vi "HART_init_address_and_MODBUS_register.vi"() -> ()   [LabVIEW 2016]
panel:
  out "Array":u16[](array[numeric])
  out "Floating pt.":sgl[](array[numeric])=[496.45227, -0.008102778, 0.0, 0.0, 0.0, 0.0, 0.0, 0.0]
  in  "Array of registers to read":T1(array[cluster])=[{"MODBUS Reg."=285, "data type"=enum."Float", "Desc."="Tube frequency"}, {"MODBUS Reg."=247, "data type"=enum."Float", "Desc."="Mass Flow"}, {"MODBUS Reg."=419, "data type"=enum."Uint16", "Desc."="Status word 1"}, {"MODBUS Reg."=420, "data type"=enum."Uint16", "Desc."="Status word 2"}, {"MODBUS Reg."=421, "data type"=enum."Uint16", "Desc."="Status word 3"}, {"MODBUS Reg."=422, "data type"=enum."Uint16", "Desc."="Status word 4"}, {"MODBUS Reg."=423, "data type"=enum."Uint16", "Desc."="Status word 5"}, {"MODBUS Reg."=424, "data type"=enum."Uint16", "Desc."="Status word 6"}]
  in  "resource name":refnum<visa-resource-name>="COM25"
  out "error out":errorcluster={"status"=FALSE, "code"=1073676294, "source"="VISA Read in HART_Read response from brooks.vi->HART_read_modbus_register.vi->HART_init_address_and_MODBUS_register.vi"}
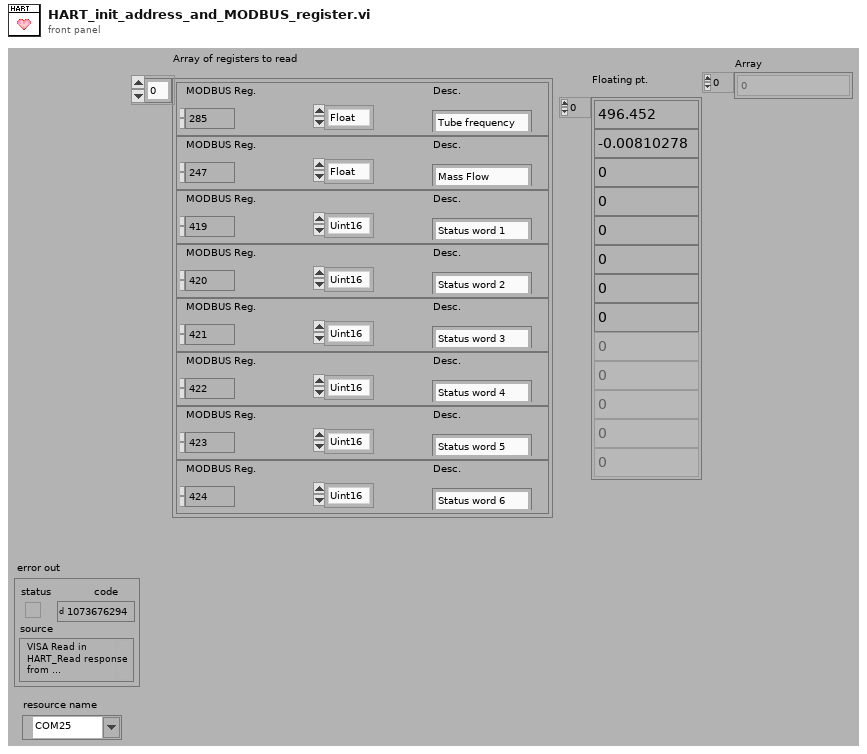
[diagram p1: front panel]
types:
  T1 = cluster{"MODBUS Reg.":u16, "data type":enum16{"None", "Coil", "Uint16", "Uint32", "Float"}, "Desc.":string}[]
  T2 = enum16{"None", "Coil", "Uint16", "Uint32", "Float"}
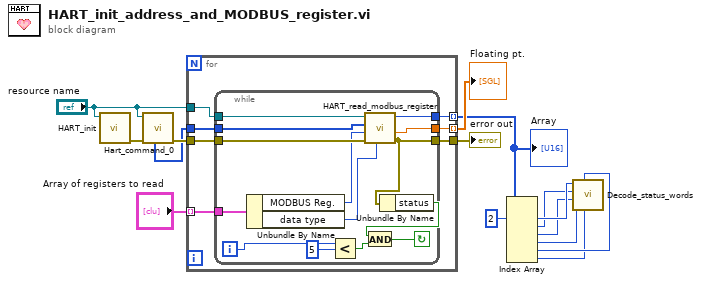
[diagram p0: block diagram]
diagram:
  n1 = call "HART_init.vi"("resource name"="resource name") -> ("error out"=w14:errorcluster)  [unwired: 10 in]
  n2 = call "Hart_command_0.vi"("error in (no error)"=w14, "VISA resource name"="resource name") -> ("error out"=w13:errorcluster, "Address (array)"=w12:u8[])  [unwired: 3 in, 5 out]
  n3 = for {
    tunnel: "resource name" -> [w22]
    tunnel: w13 -> [w21]
    tunnel: w12 -> [w20]
    tunnel: [w19] -> w11
    tunnel: [w18] -> w9 mode=indexing
    tunnel: "Array of registers to read" -> [w17] mode=indexing
    tunnel: [w16] -> w8 mode=indexing
    n4 = while {
      tunnel: w22 -> [w36]
      tunnel: w21 -> [w35]
      tunnel: w20 -> [w34]
      tunnel: [w29] -> w19
      tunnel: [w33] -> w18
      tunnel: w17 -> [w32]
      tunnel: [w23] -> w16
      i -> [w28]
      stop <- w24 continue-if-true
      n5 = Unbundle By Name(w32) -> ("MODBUS Reg."=w31:u16, "data type"=w30:T2)
      n6 = Less?(x=w28, y=5) -> (x < y?=w26:bool)
      n7 = call "HART_read_modbus_register.vi"("data type"=w30, "error IN"=w35, "MODBUS Reg."=w31, "address (array)"=w34, "port number"=w36) -> ("error out"=w29:errorcluster, "floating point out"=w33:sgl, "Unsigned 16 out"=w23:u16)  [unwired: 2 in, 2 out]
      n8 = Unbundle By Name(w29) -> ("status"=w25:bool)
      n9 = And(x=w25, y=w26) -> (x .and. y?=w24:bool)
    }
  }
  "error out" <- w11
  "Floating pt." <- w9
  "Array" <- w8
  n10 = Index Array(array=w8, index #1=2 ("index")) -> (element #1=w7:u16, element #2=w6:u16, element #3=w5:u16, element #4=w4:u16, element #5=w3:u16, element #6=w2:u16)  [unwired: 5 in]
  n11 = call "Decode_status_words.vi"("status word in 6"=w2, "status word in 5"=w3, "status word in 4"=w4, "status word in 3"=w5, "status word in 2"=w6, "status word in 1"=w7) -> ()  [unwired: 6 in]
